vi "Example 5 - Bus-ception.vi"() -> ()   [LabVIEW 2021]
uses:
  Omni-Bus/Support/Broad Types.ctl
  Aggregator Bus/Aggregator Bus.lvclass
  C:/Users/Tim/Documents/GitHub/Omni-Bus/Source/Omni-Bus/Bus Access/Bus_Access.lvclass
  Omni-Bus/Omni_Bus.lvclass
  C:/Program Files (x86)/National Instruments/LabVIEW 2021/vi.lib/TSA/Abstract Data Classes/Abs_Types/Type/Abs_Type.lvclass
  Local Bus/Local Bus.lvclass
  <vilib>/Utility/Data Type/Type Definitions/Data Type.ctl
  Omni-Bus/Support/Write/Write String.vi
  Omni-Bus/Support/Read/Read String.vi
  <vilib>/TSA/Abstract Data Classes/Abs_Types/String/Abs_String.lvclass
  <vilib>/Utility/Data Type/NI_Data Type.lvlib
panel:
  out "BUS C error out":errorcluster
  out "BUS B error out":errorcluster
  out "BUS A error out":errorcluster
  out "error out":errorcluster
  in  "BUS C Read StringTag":string
  out "BUS C String":string
  in  "BUS B Read StringTag":string
  out "BUS B String":string
  in  "BUS A Read StringTag":string
  out "BUS A String":string
  out "String":string
  in  "Read StringTag":string
  in  "Write String Tag":string
  in  "String":string
  out "Write String error":errorcluster
  in  "BUS C Write String Tag":string
  in  "BUS C String":string
  out "BUS C Write String error":errorcluster
  in  "BUS B Write String Tag":string
  in  "BUS B  String":string
  out "BUS B Write String error":errorcluster
  in  "BUS A Write String Tag":string
  in  "BUS A String":string
  out "BUS A Write String error":errorcluster
  in  "stop":bool
  out "All Tags":string[](array[string])
  # "Values are not the only\ntypes that can be accessed over the\nOmni-bus"
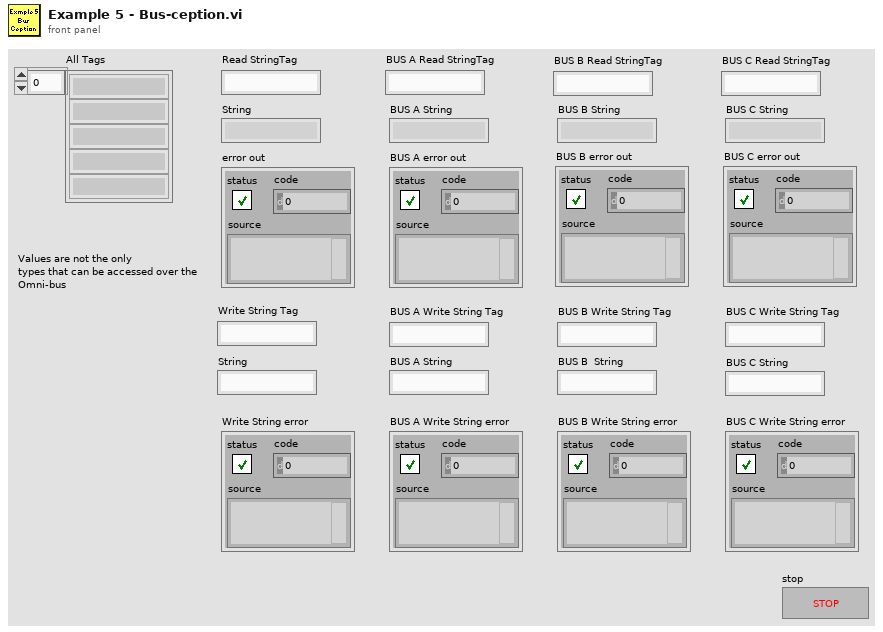
[diagram p1: front panel]
types:
  T1 = typedef "NI_Data Type.lvlib/Data Type.ctl" = enum8{"Invalid Type", "Void", "I8", "I16", "I32", "I64", "U8", "U16", "U32", "U64", "Single Float", "Double Float", "Extended Float", "Single Complex", "Double Complex", "Extended Complex", "Enum U8", "Enum U16", "Enum U32", "Enum U64", "Single Float With Unit", "Double Float With Unit", "Extended Float With Unit", "Single Complex with Unit", "Double Complex with Unit", "Extended Complex with Unit", "Boolean", "String", "Path", "Picture", "Tag", "Array", "Cluster", "Variant", "LV Variant", "Waveform", "Timestamp", "Digital Waveform", "Digital Data", "ExpressData", "Refnum", "External Data", "VI", "Poly VI", "LabVIEW Class Instance", "Fixed Point", "Set Collection", "Map Collection"}
  T2 = typedef "Omni_Bus.lvclass/Broad Types.ctl" = enum16{"All Tags", "NI Specific Type", "Boolean", "String", "Numeric", "Float", "Integer", "Collection", "All Value Types", "Non Value Types"}
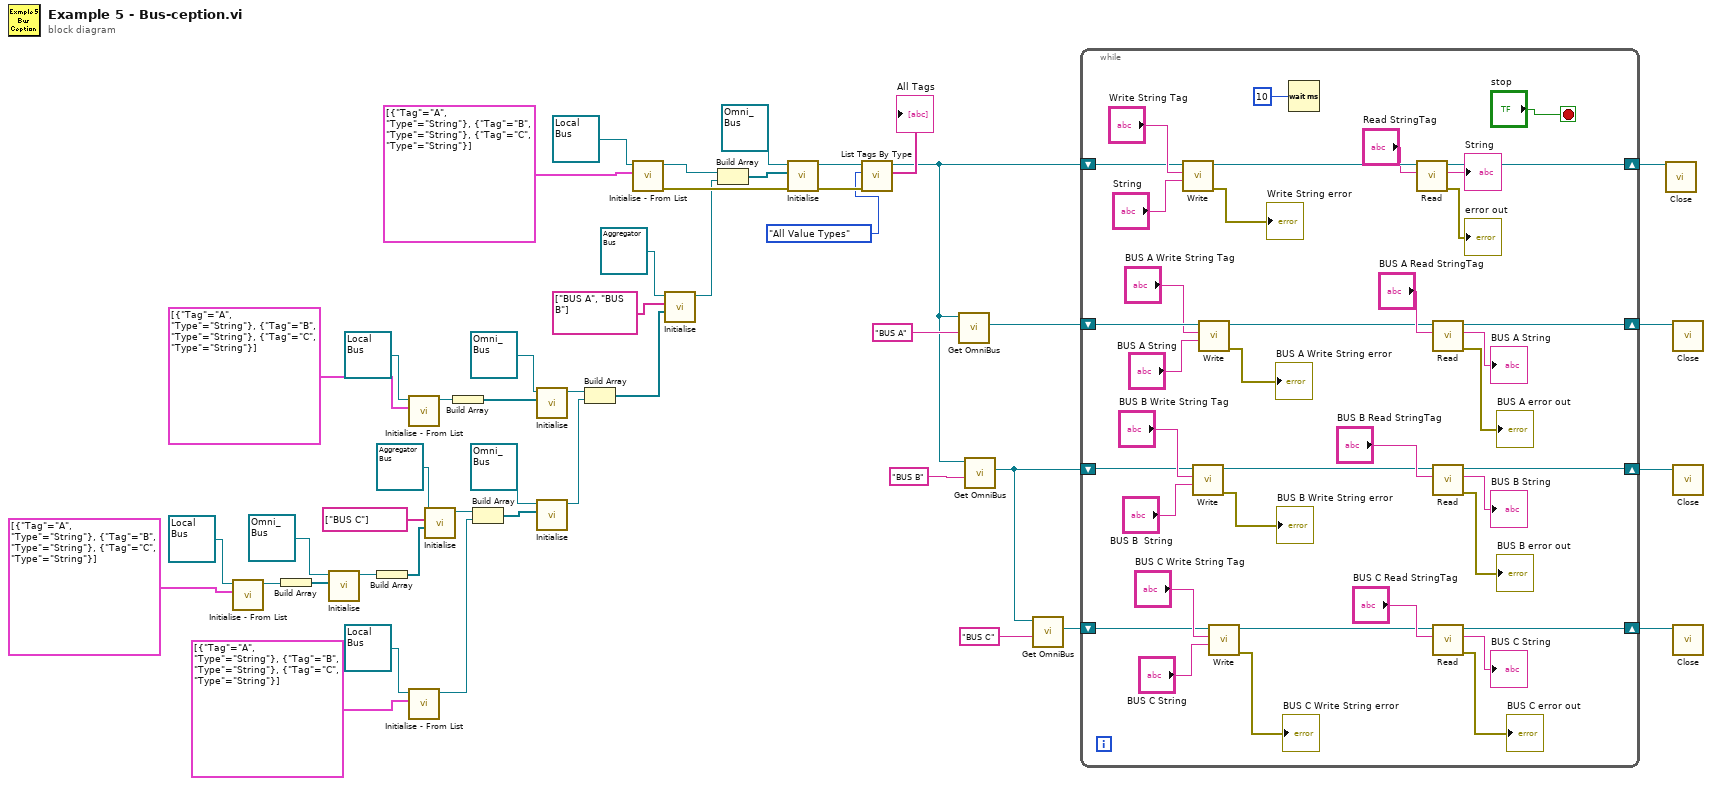
[diagram p0: block diagram]
diagram:
  n1 = call "Initialise - From List.vi"("Tag List"=cluster{"Tag":string, "Type":T1}[] [{"Tag"="A", "Type"=enum."String"}, {"Tag"="B", "Type"=enum."String"}, {"Tag"="C", "Type"=enum."String"}], "Local Bus in"=refnum<class "Local Bus.lvclass"> refnum ("Local Bus.lvclass")) -> ("Local Bus out"=w4:refnum<class "Local Bus.lvclass">)  [unwired: 8 in, 1 out]
  n2 = Build Array(w4) -> (w27:refnum<class "Local Bus.lvclass">[])
  n3 = call-dynamic "Initialise.vi"("Bus Access"=w27, "Var Bus in"=refnum<class "Omni_Bus.lvclass"> refnum) -> ("Var Bus out"=w25:refnum<class "Omni_Bus.lvclass">)  [unwired: 8 in, 1 out]
  n4 = Build Array(w25) -> (w24:refnum<class "Omni_Bus.lvclass">[])
  n5 = call "Initialise - From List.vi"("Tag List"=cluster{"Tag":string, "Type":T1}[] [{"Tag"="A", "Type"=enum."String"}, {"Tag"="B", "Type"=enum."String"}, {"Tag"="C", "Type"=enum."String"}], "Local Bus in"=refnum<class "Local Bus.lvclass"> refnum ("Local Bus.lvclass")) -> ("Local Bus out"=w8:refnum<class "Local Bus.lvclass">)  [unwired: 8 in, 1 out]
  n6 = call "Initialise - From List.vi"("Tag List"=cluster{"Tag":string, "Type":T1}[] [{"Tag"="A", "Type"=enum."String"}, {"Tag"="B", "Type"=enum."String"}, {"Tag"="C", "Type"=enum."String"}], "Local Bus in"=refnum<class "Local Bus.lvclass"> refnum ("Local Bus.lvclass")) -> ("Local Bus out"=w1:refnum<class "Local Bus.lvclass">)  [unwired: 8 in, 1 out]
  n7 = call "Initialise.vi"("Values"=w24, "Tags"=string[] ["BUS C"], "Aggregator Bus in"=refnum<class "Aggregator Bus.lvclass"> refnum) -> ("Aggregator Bus out"=w28:refnum<class "Aggregator Bus.lvclass">)  [unwired: 7 in, 1 out]
  n8 = Build Array(w8) -> (w7:refnum<class "Local Bus.lvclass">[])
  n9 = Build Array(w28, w1) -> (w29:refnum<class "Bus_Access.lvclass">[])
  n10 = call-dynamic "Initialise.vi"("Bus Access"=w7, "Var Bus in"=refnum<class "Omni_Bus.lvclass"> refnum) -> ("Var Bus out"=w21:refnum<class "Omni_Bus.lvclass">)  [unwired: 8 in, 1 out]
  n11 = call-dynamic "Initialise.vi"("Bus Access"=w29, "Var Bus in"=refnum<class "Omni_Bus.lvclass"> refnum) -> ("Var Bus out"=w20:refnum<class "Omni_Bus.lvclass">)  [unwired: 8 in, 1 out]
  n12 = Build Array(w21, w20) -> (w35:refnum<class "Omni_Bus.lvclass">[])
  n13 = call "Initialise - From List.vi"("Tag List"=cluster{"Tag":string, "Type":T1}[] [{"Tag"="A", "Type"=enum."String"}, {"Tag"="B", "Type"=enum."String"}, {"Tag"="C", "Type"=enum."String"}], "Local Bus in"=refnum<class "Local Bus.lvclass"> refnum ("Local Bus.lvclass")) -> ("error out"=w41:errorcluster, "Local Bus out"=w40:refnum<class "Local Bus.lvclass">)  [unwired: 8 in]
  n14 = call "Initialise.vi"("Values"=w35, "Tags"=string[] ["BUS A", "BUS B"], "Aggregator Bus in"=refnum<class "Aggregator Bus.lvclass"> refnum) -> ("Aggregator Bus out"=w37:refnum<class "Aggregator Bus.lvclass">)  [unwired: 7 in, 1 out]
  n15 = Build Array(w40, w37) -> (w46:refnum<class "Bus_Access.lvclass">[])
  n16 = call-dynamic "Initialise.vi"("error in (no error)"=w41, "Bus Access"=w46, "Var Bus in"=refnum<class "Omni_Bus.lvclass"> refnum) -> ("error out"=w44:errorcluster, "Var Bus out"=w45:refnum<class "Omni_Bus.lvclass">)  [unwired: 7 in]
  n17 = call-dynamic "List Tags By Type.vi"("error in (no error)"=w44, "Broad Types"=Broad_Types."All Value Types", "Var Bus in"=w45) -> ("Tags"=→"All Tags":string[], "Var Bus out"=w13:refnum<class "Omni_Bus.lvclass">)  [unwired: 5 in, 2 out]
  n18 = call-dynamic "Get OmniBus.vi"("Tag"="BUS A", "Var Bus in"=w13) -> ("Value Out"=w19:refnum<class "Omni_Bus.lvclass">)  [unwired: 7 in, 2 out]
  n19 = call-dynamic "Get OmniBus.vi"("Tag"="BUS B", "Var Bus in"=w13) -> ("Value Out"=w14:refnum<class "Omni_Bus.lvclass">)  [unwired: 7 in, 2 out]
  n20 = call-dynamic "Get OmniBus.vi"("Tag"="BUS C", "Var Bus in"=w14) -> ("Value Out"=w18:refnum<class "Omni_Bus.lvclass">)  [unwired: 7 in, 2 out]
  n21 = while {
    shift-right: [w56] -> w11
    shift-left: w19 -> [w85]
    shift-right: [w57] -> w10
    shift-left: w14 -> [w77]
    shift-right: [w52] -> w9
    shift-left: w18 -> [w73]
    shift-right: [w66] -> w12
    shift-left: w13 -> [w69]
    stop <- "stop" stop-if-true
    n22 = call-poly "Write.vi"("String"="String", "Tag"="Write String Tag", "Omni_Bus in"=w69) -> ("error out"=→"Write String error":errorcluster, "Omni_Bus out"=w67:refnum<class "Omni_Bus.lvclass">)  [unwired: 7 in]
    n23 = call-poly "Write.vi"("String"="BUS B  String", "Tag"="BUS B Write String Tag", "Omni_Bus in"=w77) -> ("error out"=→"BUS B Write String error":errorcluster, "Omni_Bus out"=w58:refnum<class "Omni_Bus.lvclass">)  [unwired: 7 in]
    n24 = call-poly "Write.vi"("String"="BUS A String", "Tag"="BUS A Write String Tag", "Omni_Bus in"=w85) -> ("error out"=→"BUS A Write String error":errorcluster, "Omni_Bus out"=w61:refnum<class "Omni_Bus.lvclass">)  [unwired: 7 in]
    n25 = call-poly "Write.vi"("String"="BUS C String", "Tag"="BUS C Write String Tag", "Omni_Bus in"=w73) -> ("error out"=→"BUS C Write String error":errorcluster, "Omni_Bus out"=w53:refnum<class "Omni_Bus.lvclass">)  [unwired: 7 in]
    n26 = Wait (ms)(milliseconds to wait=u32 10) -> ()  [unwired: 1 out]
    n27 = call-poly "Read.vi"("Tag"="Read StringTag", "Var Bus in"=w67) -> ("error out"=→"error out":errorcluster, "String"=→"String":string, "Var Bus out"=w66:refnum<class "Omni_Bus.lvclass">)  [unwired: 7 in]
    n28 = call-poly "Read.vi"("Tag"="BUS A Read StringTag", "Var Bus in"=w61) -> ("error out"=→"BUS A error out":errorcluster, "String"=→"BUS A String":string, "Var Bus out"=w56:refnum<class "Omni_Bus.lvclass">)  [unwired: 7 in]
    n29 = call-poly "Read.vi"("Tag"="BUS B Read StringTag", "Var Bus in"=w58) -> ("error out"=→"BUS B error out":errorcluster, "String"=→"BUS B String":string, "Var Bus out"=w57:refnum<class "Omni_Bus.lvclass">)  [unwired: 7 in]
    n30 = call-poly "Read.vi"("Tag"="BUS C Read StringTag", "Var Bus in"=w53) -> ("error out"=→"BUS C error out":errorcluster, "String"=→"BUS C String":string, "Var Bus out"=w52:refnum<class "Omni_Bus.lvclass">)  [unwired: 7 in]
  }
  n31 = call-dynamic "Close.vi"("Data in"=w12) -> ()  [unwired: 9 in, 2 out]
  n32 = call-dynamic "Close.vi"("Data in"=w11) -> ()  [unwired: 9 in, 2 out]
  n33 = call-dynamic "Close.vi"("Data in"=w10) -> ()  [unwired: 9 in, 2 out]
  n34 = call-dynamic "Close.vi"("Data in"=w9) -> ()  [unwired: 9 in, 2 out]
